vi "IBM4_Read(Ave).vi"(8 "error in":errorcluster, 9 "Averages":i32=10 min=1, 10 "Channel":enum16{"A2", "A3", "A4", "A5"}(ring), 11 "COM resource in":refnum<visa-resource-name>="ASRL5::INSTR") -> (0 "error out":errorcluster, 2 "output":dbl=1.85786, 3 "COM resource out":refnum<visa-resource-name>="ASRL5::INSTR")   [LabVIEW 2023, in "IBM4.lvlib"]
doc: "This VI interfaces with the IBM4 to perform a read operation.\n\nThe number of readings should be greater than zero. At some point the number of reading will be too high and will cause a timeout error. This should only happen for numbers larger than 10000. The output will be a single Voltage (floating point) value representing the average of the multiple readings.\n\nAlternate read operations exist covering binary or floating point, single reading, multiple readings, and an average of multiple readings (floating point only)."
uses:
  <instrlib>/IBM4/IBM4.lvlib
panel:
  out "read buffer":string="Output 3 = 1.85786 \r\n"
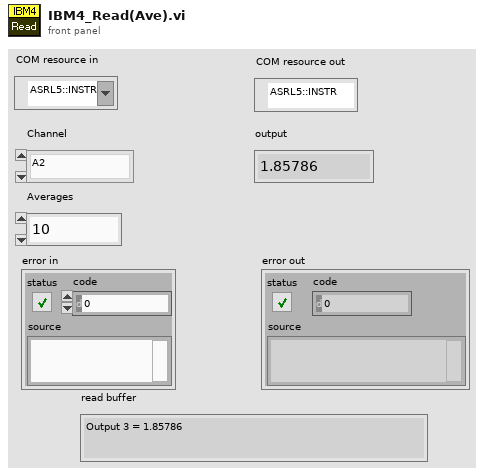
[diagram p1: front panel]
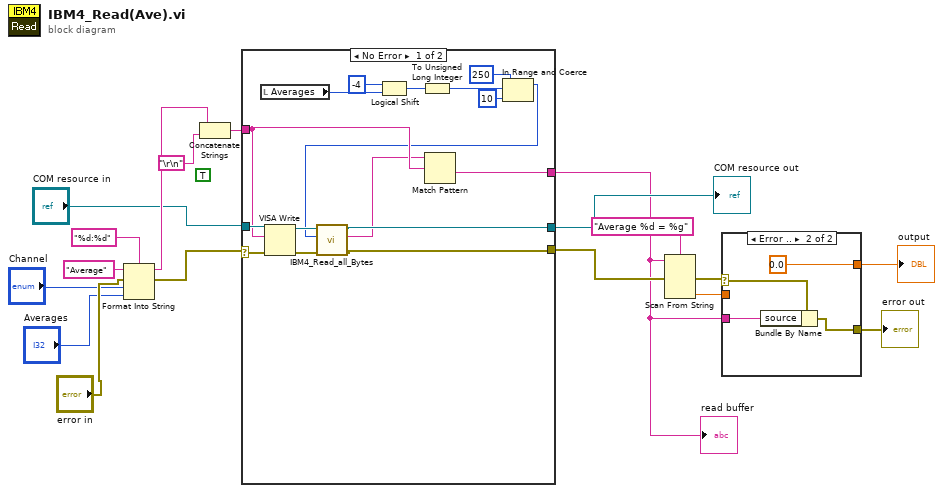
[diagram p0: block diagram]
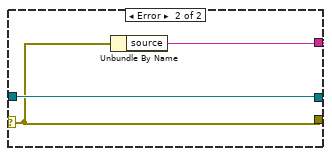
[diagram p3: hidden frame]
diagram:
  (unwired) TRUE ("Enable Termination\nChar (T)")
  n1 = Format Into String(format string="%d:%d", initial string="Average", error in="error in", "Channel", "Averages") -> (resulting string=w10:string, error out=w2:errorcluster)
  n2 = Concatenate Strings(w10, "\r\n") -> (w9:string)
  n3 = case shown="No Error" w2 {
    selector: w2 -> [w31 w35]
    tunnel: "COM resource in" -> [w34 w37]
    tunnel: [w20 w35] -> w13
    tunnel: [w33 w36] -> w4
    tunnel: w9 -> [w32 _]
    tunnel: [w21 w37] -> w14
    frame No Error {
      n4 = local read "Averages"() -> (w23:i32)
      n5 = VISA Write(VISA resource name=w34, write buffer=w32, error in (no error)=w31) -> (VISA resource name out=w30:refnum<visa-resource-name>, error out=w29:errorcluster)  [unwired: 1 out]
      n6 = Logical Shift(y=i16 -4, x=w23) -> (x << y=w26:i32)
      n7 = To Unsigned Long Integer(number=w26) -> (unsigned 32bit integer=w24:u32)
      n8 = In Range and Coerce(upper limit=u32 250, x=w24, lower limit=u32 10) -> (coerced(x)=w22:u32)  [unwired: 1 out]
      n9 = call <instrlib>:"IBM4_Read_all_Bytes.vi"("error in (no error)"=w29, "milliseconds to wait"=w22, "VISA Refnum in"=w30) -> ("error out"=w20:errorcluster, "String"=w19:string, "VISA Refnum out"=w21:refnum<visa-resource-name>)  [unwired: 2 in]
      n10 = Match Pattern(string=w19, regular expression=w32) -> (after substring=w33:string)  [unwired: 1 in, 3 out]
    }
    frame Error {
      n11 = Unbundle By Name(w35) -> ("source"=w36:string)
    }
  }
  "COM resource out" <- w14
  "read buffer" <- w4
  n12 = Scan From String(format string="Average %d = %g", input string=w4, error in=w13) -> (error out=w8:errorcluster, output 2=w7:dbl)  [unwired: 4 in, 2 out]
  n13 = case shown="Error .." w8 {
    selector: w8 -> [w38 w42]
    tunnel: w7 -> [w39 _]
    tunnel: [w39 0.0] -> w6
    tunnel: [w38 w40] -> w5
    tunnel: w4 -> [_ w41]
    frame No Error {
    }
    frame Error {
      n14 = Bundle By Name(cluster=w42, "source"=w41) -> (w40:errorcluster)
    }
  }
  "error out" <- w5
  "output" <- w6
